vi "AlliGator Load Single HDF5 Gate Image v 0.3b.vi"(6 "Action":T1, 8 "error in (no error)":errorcluster, 10 "File Info":variant, 11 "Gate Index":i32) -> (0 "error out":errorcluster, 1 "Data 2":sgl[][](array[numeric]), 3 "Data 1":sgl[][](array[numeric]))   [LabVIEW 2021, in "AlliGator HDF5.lvlib"]
doc: "Loads single gate image (or dual-channel images) from HDF5 FLI dataset file (v0.3b)."
uses:
  AlliGator HDF5.lvlib
  AlliGator FLI Image Stack Action.ctl
  AlliGator HDF5 FLI File Loading Information v0.6.ctl
  <vilib>/addons/h5labview2/base/lib_path.vi
  <vilib>/addons/h5labview2/base/H5Equery.vi
  <vilib>/Utility/error.llb/Error Cluster From Error Code.vi
  <vilib>/addons/h5labview2/base/hid_t.ctl
  <vilib>/addons/h5labview2/dataset/H5Dread.llb/H5Dread.xnode
  <vilib>/ErrorRing/Error Ring.xnode
  <vilib>/addons/h5labview2/file/H5F.lvlib
  <vilib>/addons/h5labview2/group/H5G.lvlib
panel:
  # "see the AlliGator License on the block diagram (Ctrl+E or Window:Show Block Diagram)"
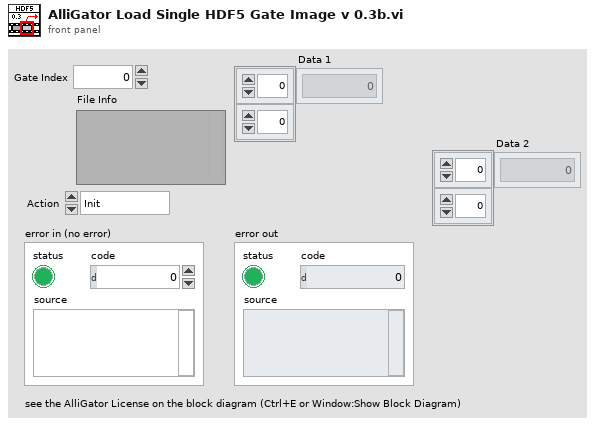
[diagram p1: front panel]
types:
  T1 = typedef "AlliGator HDF5.lvlib/AlliGator FLI Image Stack Action.ctl" = enum16{"Init", "Get Image", "Close"}
  T2 = typedef "AlliGator HDF5.lvlib/AlliGator HDF5 FLI File Loading Information v0.6.ctl" = cluster{"HDF5 File Path":path, "Data Type":string, "# Datasets in Series":i32, "Dataset ID in Series":i32, "Channel Names":string[]}
  T3 = typedef "hid_t.ctl" = i64
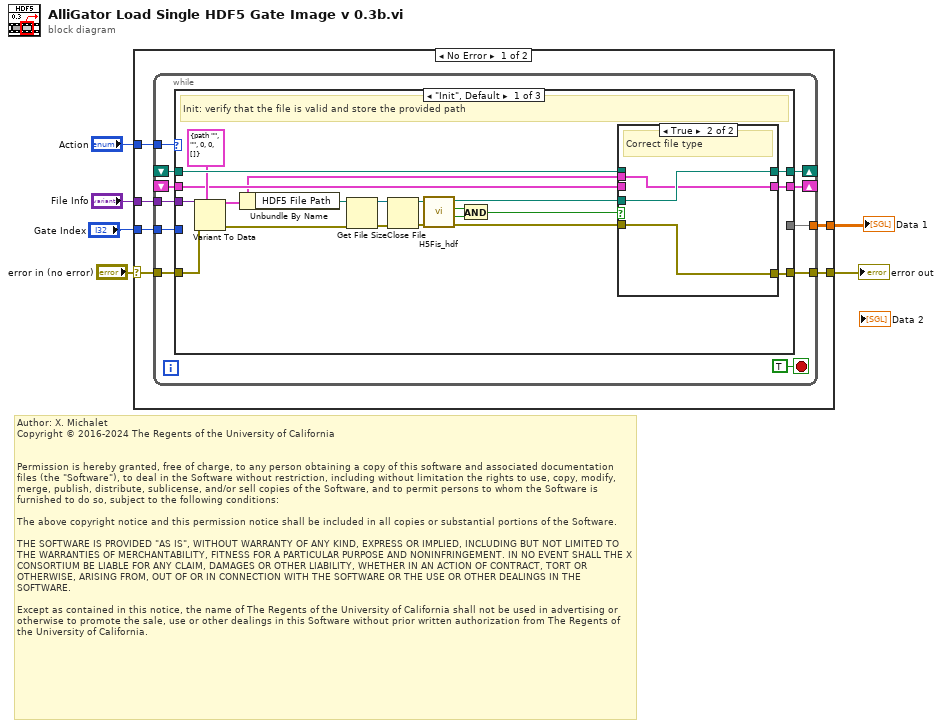
[diagram p0: block diagram]
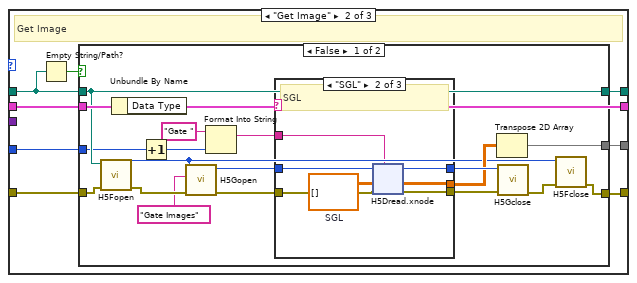
[diagram p3: hidden frame]
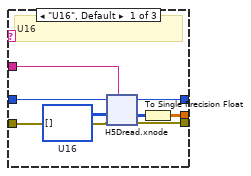
[diagram p4: hidden frame]
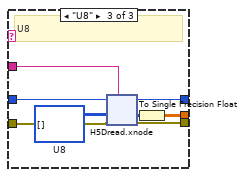
[diagram p5: hidden frame]
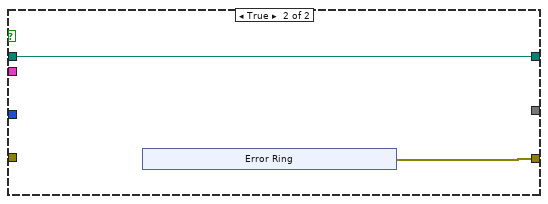
[diagram p6: hidden frame]
diagram:
  # "Author: X. Michalet\nCopyright © 2016-2024 The Regents of the University of California\n \n\nPermission is hereby granted, free of charge, to any person obtaining a copy of this software and associated documentation files (the \"Software\"), to deal in the Software without restriction, including without limitation the rights to use, copy, modify, merge, publish, distribute, sublicense, and/or sell copies of the Software, and to permit persons to whom the Software is furnished to do so, subject to the following conditions:\n\nThe above copyright notice and this permission notice shall be included in all copies or substantial portions of the Software.\n\nTHE SOFTWARE IS PROVIDED \"AS IS\", WITHOUT WARRANTY OF ANY KIND, EXPRESS OR IMPLIED, INCLUDING BUT NOT LIMITED TO THE WARRANTIES OF MERCHANTABILITY, FITNESS FOR A PARTICULAR PURPOSE AND NONINFRINGEMENT. IN NO EVENT SHALL THE X CONSORTIUM BE LIABLE FOR ANY CLAIM, DAMAGES OR OTHER LIABILITY, WHETHER IN AN ACTION OF CONTRACT, TORT OR OTHERWISE, ARISING FROM, OUT OF OR IN CONNECTION WITH THE SOFTWARE OR THE USE OR OTHER DEALINGS IN THE SOFTWARE.\n\nExcept as contained in this notice, the name of The Regents of the University of California shall not be used in advertising or otherwise to promote the sale, use or other dealings in this Software without prior written authorization from The Regents of the University of California."
  n1 = case shown="No Error" "error in (no error)" {
    selector: "error in (no error)" -> [w11 w152]
    tunnel: [w10 w152] -> w5
    tunnel: "Action" -> [w12 _]
    tunnel: "File Info" -> [w9 _]
    tunnel: "Gate Index" -> [w8 _]
    tunnel: [w7 _] -> w1
    frame No Error {
      n2 = while {
        tunnel: w12 -> [w22]
        tunnel: w11 -> [w21]
        tunnel: [w20] -> w10
        tunnel: w9 -> [w19]
        shift-right: [w18] -> _
        shift-left: _ -> [w17]
        tunnel: w8 -> [w16]
        tunnel: [w15] -> w7
        shift-right: [w14] -> _
        shift-left: _ -> [w13]
        stop <- TRUE stop-if-true
        n3 = case shown="\"Init\", Default" w22 {
          tunnel: w21 -> [w30 w53 w151]
          tunnel: [w32 w56 w151] -> w20
          tunnel: w19 -> [w31 _ _]
          tunnel: [w34 w57 _] -> w18
          tunnel: w17 -> [w33 w55 _]
          tunnel: w16 -> [_ w52 _]
          tunnel: [_ w51 _] -> w15
          tunnel: [w26 w50 _] -> w14
          tunnel: w13 -> [w25 w50 _]
          frame "Init", Default {
            # "Init: verify that the file is valid and store the provided path"
            n4 = Variant To Data(error in=w30, type=T2 {"HDF5 File Path"=path "", "Data Type"="", "# Datasets in Series"=0, "Dataset ID in Series"=0, "Channel Names"=[]} ("HDF5 FLI File Loading Information"), Variant=w31) -> (data=w24:T2, error out=w28:errorcluster)
            n5 = Unbundle By Name(w24) -> ("HDF5 File Path"=w27:path)
            n6 = Get File Size(file=w27, error in=w28) -> (refnum out=w40:refnum<file>, 0:w41:errorcluster)  [unwired: 1 out]
            n7 = Close File(refnum=w40, error in=w41) -> (path=w39:path, error out=w38:errorcluster)
            n8 = call <vilib>:"H5Fis_hdf.vi"("error in (no error)"=w38, "path in"=w39) -> ("error out"=w36:errorcluster, "valid?"=w42:bool, "exists?"=w43:bool, "path out"=w35:path)  [unwired: 6 in]
            n9 = And(x=w43, y=w42) -> (x .and. y?=w37:bool)
            n10 = case shown="True" w37 {
              tunnel: w36 -> [w45 w48]
              tunnel: w35 -> [_ w49]
              tunnel: [w46 w49] -> w34
              tunnel: w33 -> [w46 _]
              tunnel: [w45 w48] -> w32
              tunnel: [w44 w47] -> w26
              tunnel: w25 -> [w44 _]
              tunnel: w24 -> [_ w47]
              frame False {
                # "not legible"
              }
              frame True {
                # "Correct file type"
              }
            }
          }
          frame "Get Image" {
            # "Get Image"
            n11 = Empty String/Path?(string/path=w55) -> (empty?=w54:bool)
            n12 = case shown="False" w54 {
              tunnel: [w71 w146] -> w57
              tunnel: w55 -> [w71 w146]
              tunnel: [w73 w145] -> w56
              tunnel: w53 -> [w72 _]
              tunnel: w52 -> [w69 _]
              tunnel: [w62 _] -> w51
              tunnel: w50 -> [w61 _]
              frame False {
                n13 = call <vilib>:"H5Fopen.vi"("error in (no error)"=w72, "path"=w71) -> ("error out"=w76:errorcluster, "ref out"=w63:T3)  [unwired: 8 in]
                n14 = Unbundle By Name(w61) -> ("Data Type"=w60:string)
                n15 = Increment(x=w69) -> (x+1=w68:i32)
                n16 = call <vilib>:"H5Gopen.vi"("error in (no error)"=w76, "name"="Gate Images", "ref in"=w63) -> ("error out"=w59:errorcluster, "group out"=w58:T3)  [unwired: 7 in]
                n17 = Format Into String(initial string="Gate ", w68) -> (resulting string=w65:string)  [unwired: 2 in, 1 out]
                n18 = case shown="\"SGL\"" w60 {
                  tunnel: w58 -> [w83 w105 w128]
                  tunnel: [w82 w104 w127] -> w67
                  tunnel: [w80 w100 w125] -> w66
                  tunnel: w65 -> [w79 w103 w124]
                  tunnel: [w78 w102 w123] -> w64
                  tunnel: w59 -> [w77 w101 w122]
                  frame "U16", Default {
                    w84 = u16[][] []  # U16
                    # "U16"
                    n19 = xnode "H5Dread.xnode"("dataset name (this)"=w79, "error in (no error)"=w77, "default"=w84, "ref in"=w83) -> ("error out"=w78:errorcluster, "data"=w81:u16[][], "ref out"=w82:T3)  [unwired: 2 in, 1 out]
                    n20 = To Single Precision Float(number=w81) -> (single precision float=w80:sgl[][])
                  }
                  frame "SGL" {
                    w106 = sgl[][] []  # SGL
                    # "SGL"
                    n21 = xnode "H5Dread.xnode"("dataset name (this)"=w103, "error in (no error)"=w101, "default"=w106, "ref in"=w105) -> ("error out"=w102:errorcluster, "data"=w100:sgl[][], "ref out"=w104:T3)  [unwired: 2 in, 1 out]
                  }
                  frame "U8" {
                    w129 = u8[][] []  # U8
                    # "U8"
                    n22 = xnode "H5Dread.xnode"("dataset name (this)"=w124, "error in (no error)"=w122, "default"=w129, "ref in"=w128) -> ("error out"=w123:errorcluster, "data"=w126:u8[][], "ref out"=w127:T3)  [unwired: 2 in, 1 out]
                    n23 = To Single Precision Float(number=w126) -> (single precision float=w125:sgl[][])
                  }
                }
                n24 = Transpose 2D Array(2D array=w66) -> (transposed array=w62:sgl[][])
                n25 = call <vilib>:"H5Gclose.vi"("error in (no error)"=w64, "group in"=w67) -> ("error out"=w74:errorcluster)  [unwired: 9 in]
                n26 = call <vilib>:"H5Fclose.vi"("error in (no error)"=w74, "ref"=w63) -> ("error out"=w73:errorcluster)  [unwired: 9 in]
              }
              frame True {
                n27 = xnode "Error Ring"() -> ("error out"=w145:errorcluster)
              }
            }
          }
          frame "Close" {
            # "Close File"
          }
        }
      }
    }
    frame Error {
    }
  }
  "Data 1" <- w1
  "error out" <- w5
